vi "UART.vi"() -> ()   [LabVIEW 2014]
uses:
  <vilib>/Instr/_visa.llb/VISA Configure Serial Port (Instr).vi
panel:
  out "decimal integer string":string
  in  "stop":bool
  in  "VISA resource name":refnum<visa-resource-name>
  out "read buffer":string
  in  "write buffer":dbl(slide) scale=1.0..9.0
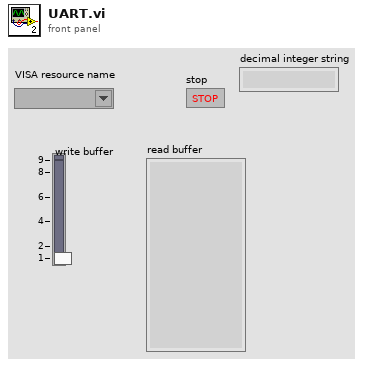
[diagram p1: front panel]
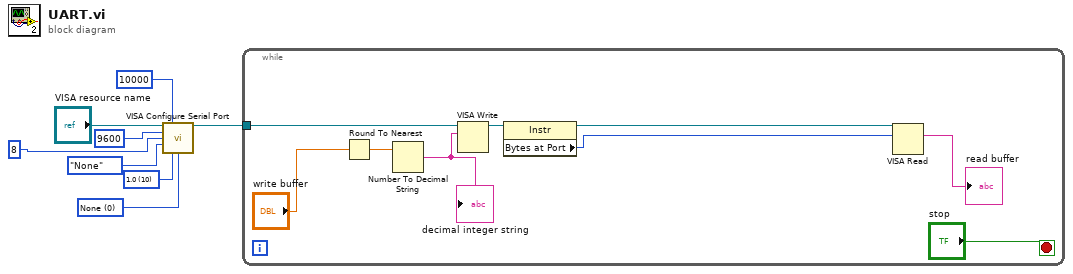
[diagram p0: block diagram]
diagram:
  w1 = u16 0 items=["None", "XON/XOFF", "RTS/CTS", "XON/XOFF & RTS/CTS", "DTR/DSR", "XON/XOFF & DTR/DSR"] ("flow control (0:none)")
  w2 = u16 10 items=["1.0"=10, "1.5"=15, "2.0"=20] ("stop bits (10: 1 bit)")
  n1 = call-poly "VISA Configure Serial Port"("VISA resource name"="VISA resource name", "timeout (10sec)"=u32 10000, "baud rate (9600)"=u32 9600, "data bits (8)"=u16 8, "parity (0:none)"=enum16{"None", "Odd", "Even", "Mark", "Space"}."None", "stop bits (10: 1 bit)"=w2, "flow control (0:none)"=w1) -> ("VISA resource name out"=w8:refnum<visa-resource-name>)  [unwired: 7 in, 1 out]
  n2 = while {
    tunnel: w8 -> [w17]
    stop <- "stop" stop-if-true
    n3 = Round To Nearest(number="write buffer") -> (nearest integer value=w10:dbl)
    n4 = Number To Decimal String(number=w10) -> (decimal integer string=w11:string)  [unwired: 1 in]
    "decimal integer string" <- w11
    n5 = VISA Write(VISA resource name=w17, write buffer=w11) -> (VISA resource name out=w16:refnum<visa-resource-name>)  [unwired: 1 in, 2 out]
    n6 = property class="Instr"(reference=w16) -> (reference out=w15:refnum<visa-resource-name>, "Bytes at Port"=w14:u32)  [unwired: 1 in, 1 out]
    n7 = VISA Read(VISA resource name=w15, byte count=w14) -> (read buffer=→"read buffer":string)  [unwired: 1 in, 3 out]
  }
